vi "energie.vi"() -> ()   [LabVIEW 2024]
uses:
  <vilib>/Analysis/baseanly.llb/Mean (DBL).vi
  EFmeter.lvlib
  <vilib>/Analysis/NI_AALBase.lvlib
  BK Precision 8500B Series/BK Precision 8500B Series.lvlib
panel:
  in  "VISA resource name":refnum<visa-resource-name>
  in  "Clear":bool
  in  "Typ zatěže":u16(ring) items=["Manualni", "BK 8542B"]
  in  "Uložit data":bool
  in  "file path (use dialog)":path
  in  "Vzorku na krokù":u16 max=100 step=1
  in  "Prumerovani":bool
  in  "start":dbl
  out "error out 2":errorcluster
  in  "velikost kroku":dbl
  in  "VISA resource name 2":refnum<visa-resource-name>
  out "Aktuální Zátěž":dbl=2.5
  in  "Prodleva mezi vzorky":u32
  out "R_out":dbl
  in  "Pocet kroku":i32
  out "XY Graph 2":cluster{"X":dbl[], "Y":dbl[]}[](graph)
  in  "stop":bool
  in  "Start":bool
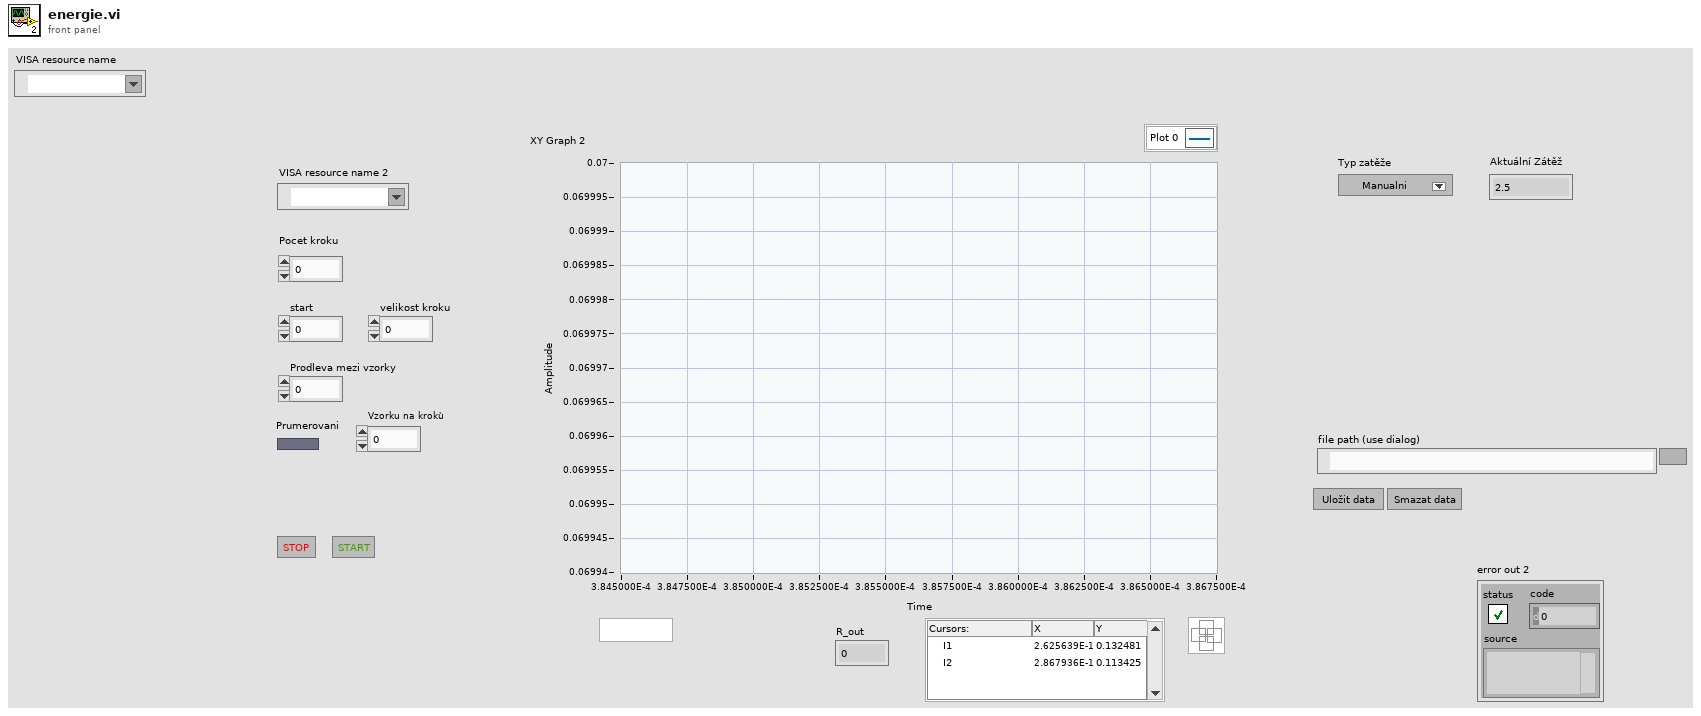
[diagram p1: front panel]
types:
  T1 = enum16{"init", "wait", "graph", "meas", "change_load", "init_measurment", "save", "clear"}
  T2 = typedef "LVCursorListTypeDef.ctl" = cluster{"Name":string, "Color":u32, "Style":u8, "Point Style":u8, "Name Visible":bool, "Allow Drag":bool, "Cursor Mode":u32, "Plot":i32, "Index":i32, "Position":cluster{"X":dbl, "Y":dbl}, "X Scale":u32, "Y Scale":u32, "Watch Plots":i32[], "Watch All Plots":bool, "Plot Area":i32, "Label Offset":cluster{"X":dbl, "Y":dbl}}[]
  T3 = cluster{"Name":string, "Color":u32, "Style":u8, "Point Style":u8, "Name Visible":bool, "Allow Drag":bool, "Cursor Mode":u32, "Plot":i32, "Index":i32, "Position":cluster{"X":dbl, "Y":dbl}, "X Scale":u32, "Y Scale":u32, "Watch Plots":i32[], "Watch All Plots":bool, "Plot Area":i32, "Label Offset":cluster{"X":dbl, "Y":dbl}}
  T4 = enum16{"open", "replace", "create", "open or create", "replace or create", "replace or create with confirmation"}
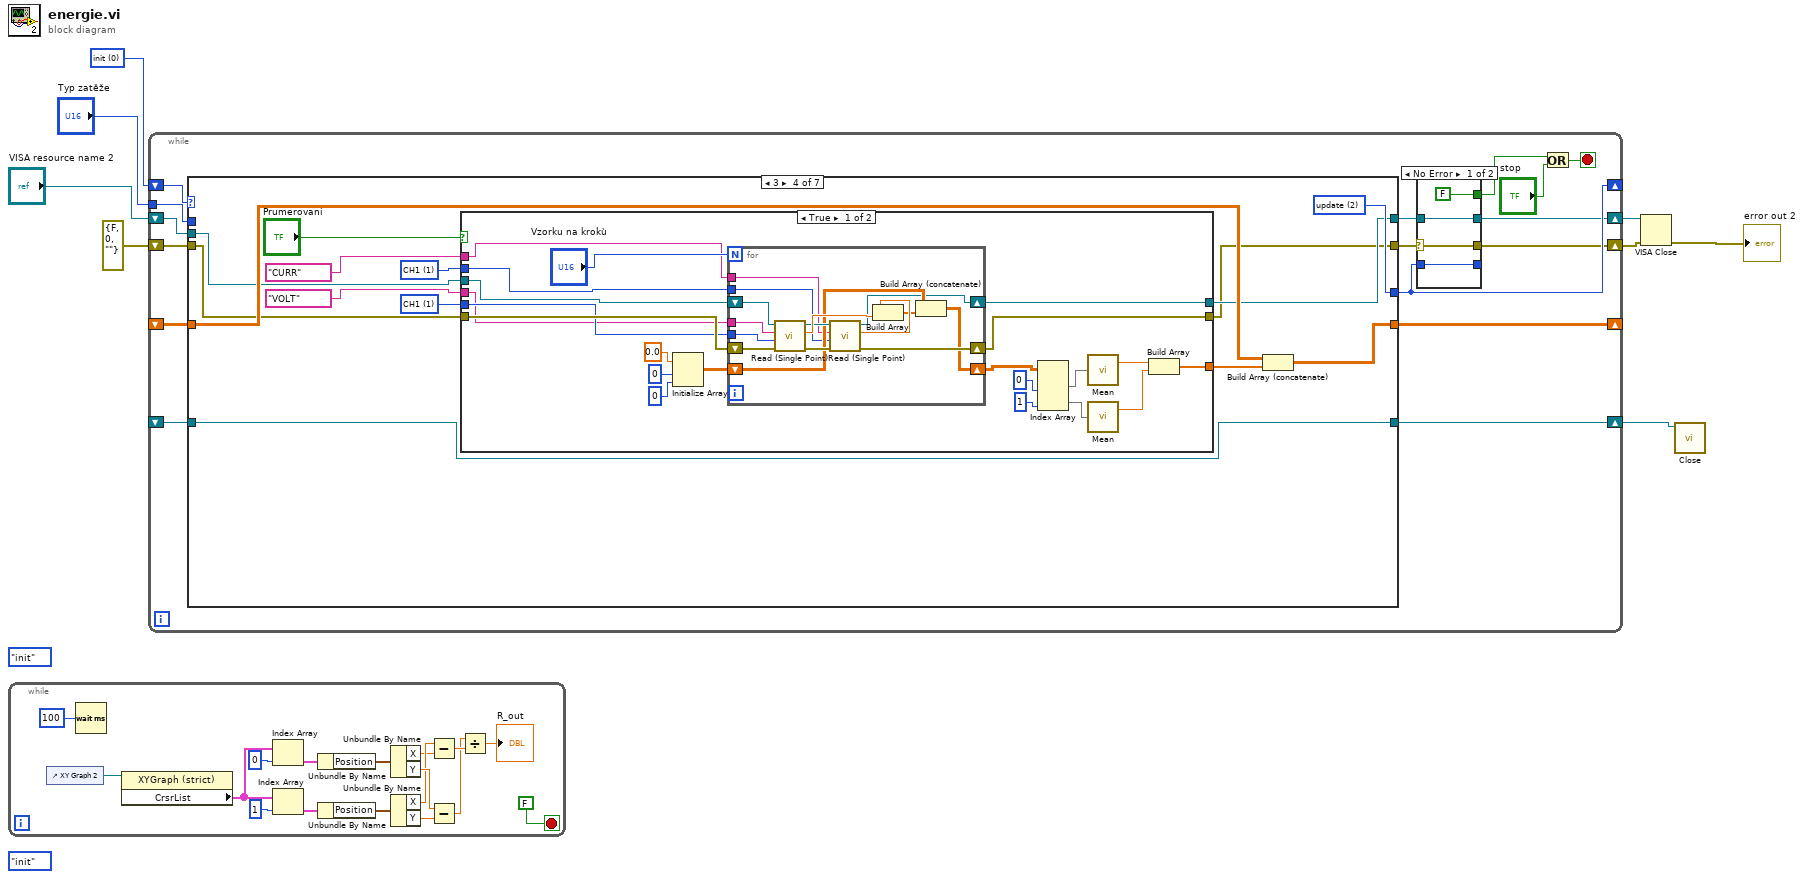
[diagram p0: block diagram]
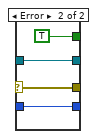
[diagram p2: hidden frame]
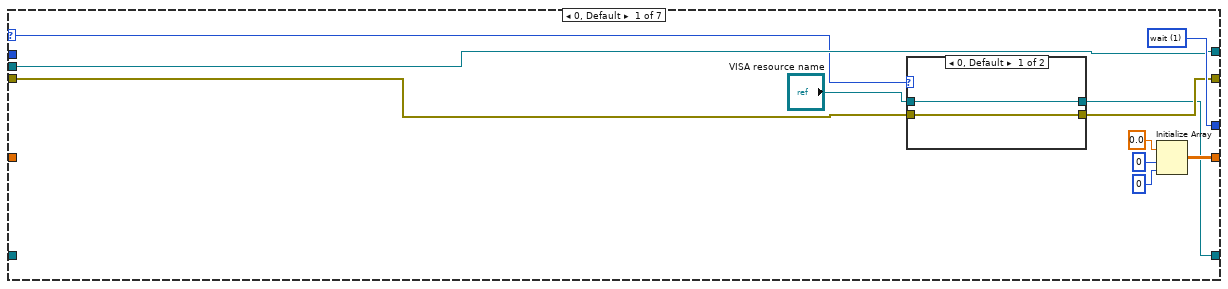
[diagram p3: hidden frame]
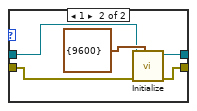
[diagram p4: hidden frame]
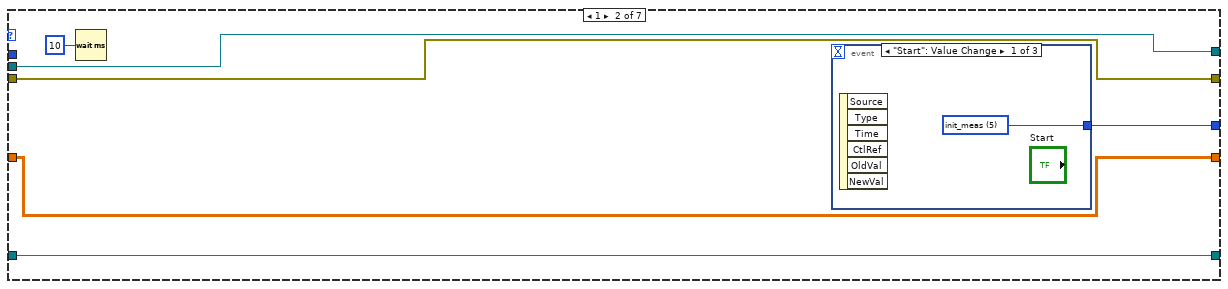
[diagram p5: hidden frame]
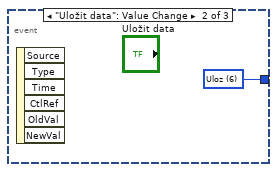
[diagram p6: hidden frame]
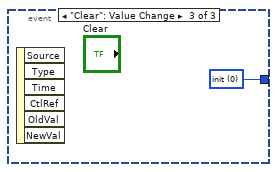
[diagram p7: hidden frame]
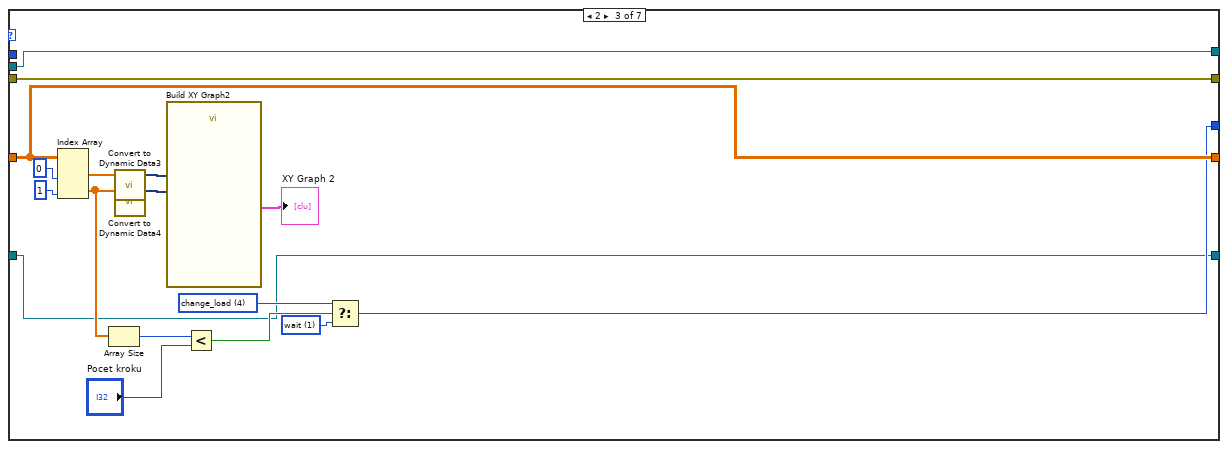
[diagram p8: hidden frame]
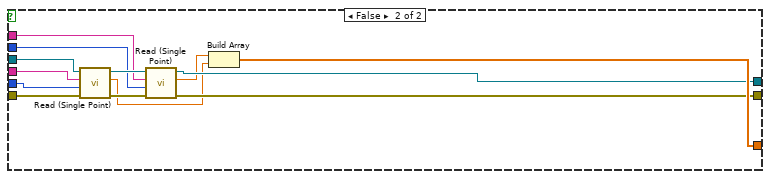
[diagram p9: hidden frame]
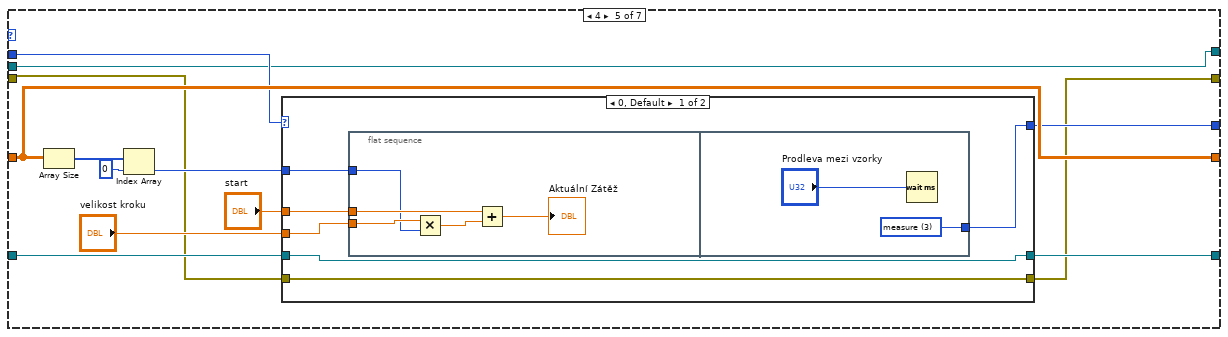
[diagram p10: hidden frame]
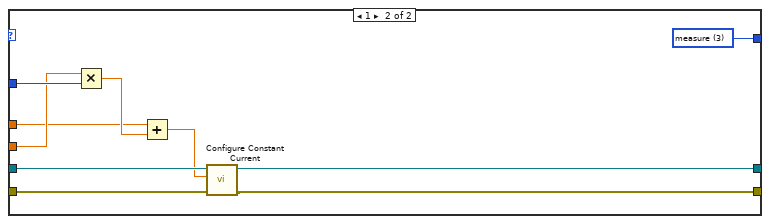
[diagram p11: hidden frame]
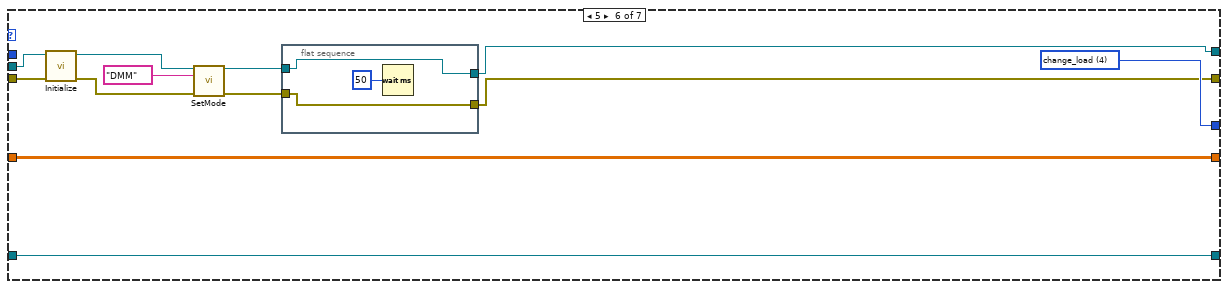
[diagram p12: hidden frame]
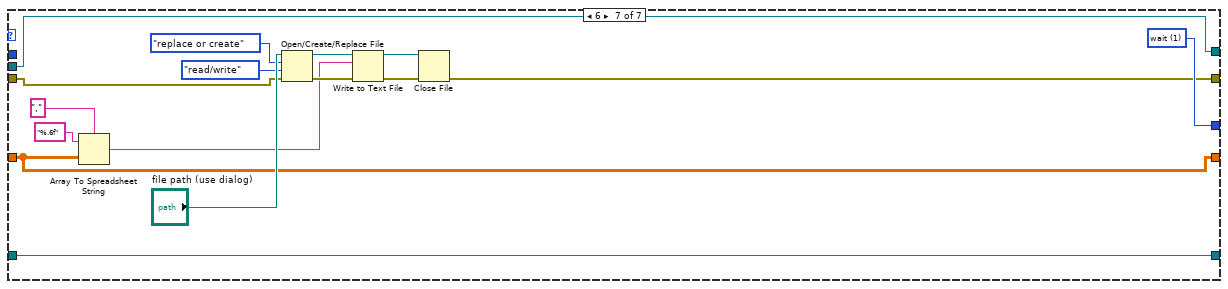
[diagram p13: hidden frame]
diagram:
  (unwired) T1."init"
  (unwired) T1."init"
  w8 = u16 0 items=["init", "wait", "update", "measure", "change_load", "init_meas", "Uloz", "clear"]
  n1 = while {
    stop <- FALSE stop-if-true
    n2 = control-ref of="XY Graph 2"() -> (w23:refnum<vi>)
    n3 = Wait (ms)(milliseconds to wait=u32 100) -> ()  [unwired: 1 out]
    n4 = property class="XYGraph (strict)"(reference=w23) -> ("CrsrList"=w18:T2)  [unwired: 1 in, 2 out]
    n5 = Index Array(array=w18, index=0) -> (element=w24:T3)
    n6 = Index Array(array=w18, index=1) -> (element=w20:T3)
    n7 = Unbundle By Name(w24) -> ("Position"=w25:cluster{"X":dbl, "Y":dbl})
    n8 = Unbundle By Name(w20) -> ("Position"=w21:cluster{"X":dbl, "Y":dbl})
    n9 = Unbundle By Name(w25) -> ("X"=w9:dbl, "Y"=w16:dbl)
    n10 = Unbundle By Name(w21) -> ("X"=w10:dbl, "Y"=w17:dbl)
    n11 = Subtract(x=w10, y=w9) -> (x-y=w12:dbl)
    n12 = Subtract(x=w16, y=w17) -> (x-y=w11:dbl)
    n13 = Divide(x=w11, y=w12) -> (x/y=→"R_out":dbl)
  }
  n14 = while {
    shift-right: [w41] -> _
    shift-left: _ -> [w40]
    shift-right: [w36] -> _
    shift-left: w8 -> [w39]
    shift-right: [w33] -> w4
    shift-left: "VISA resource name 2" -> [w38]
    shift-right: [w32] -> w3
    shift-left: errorcluster {"status"=FALSE, "code"=0, "source"=""} ("error in (no error)") -> [w37]
    tunnel: "Typ zatěže" -> [w28]
    shift-right: [w27] -> w1
    shift-left: _ -> [w26]
    stop <- w30 stop-if-true
    n15 = case shown="3" w39 {
      selector: w39 -> [w54 _ _ _ _ _ _]
      tunnel: [w58 w72 w85 w106 w169 w204 w218] -> w41
      tunnel: w40 -> [_ w72 w85 w107 w169 w204 w218]
      tunnel: [w57 w73 w84 w104 w167 w198 w216] -> w36
      tunnel: [w52 w70 w78 w96 w157 w195 w212] -> w35
      tunnel: [w55 w71 w79 w97 w166 w197 w223] -> w34
      tunnel: w38 -> [w55 w71 w79 w103 w166 w200 w223]
      tunnel: w37 -> [w53 w70 w78 w102 w158 w199 w219]
      tunnel: w28 -> [_ _ _ _ w168 _ _]
      tunnel: [w51 w68 w77 w94 w164 w193 w208] -> w27
      tunnel: w26 -> [_ w68 w77 w94 w165 w193 w208]
      frame 0, Default {
        w57 = u16 1 items=["init", "wait", "update", "measure"]
        n16 = case shown="0, Default" w54 {
          tunnel: w53 -> [w62 w66]
          tunnel: [w62 w65] -> w52
          tunnel: [w61 w64] -> w51
          tunnel: "VISA resource name" -> [w61 w63]
          frame 0, Default {
          }
          frame 1 {
            n17 = call "Initialize.vi"("Serial Configuration"=cluster{"Baud Rate":u32} {"Baud Rate"=9600}, "error in (no error)"=w66, "VISA resource name"=w63) -> ("error out"=w65:errorcluster, "VISA resource name out"=w64:refnum<visa-resource-name>)  [unwired: 7 in]
          }
        }
        n18 = Initialize Array(0.0 ("element"), 0 ("dimension size"), 0 ("dimension size")) -> (w58:dbl[][])
      }
      frame 1 {
        n19 = Wait (ms)(milliseconds to wait=u32 10) -> ()  [unwired: 1 out]
        n20 = event shown="[0] \"Start\": Value Change" {
          selector: _ -> [_ _ _]
          dyn-events: _ -> [_ _ _]
          timeout: _ -> [_ _ _]
          tunnel: [w74 w75 w76] -> w73
          event "Start": Value Change {
            w74 = u16 5 items=["init", "wait", "update", "measure", "change_load", "init_meas"]
            n21 = event-data() -> ()  [unwired: 1 in, 6 out]
          }
          event "Uložit data": Value Change {
            w75 = u16 6 items=["init", "wait", "update", "measure", "change_load", "init_meas", "Uloz"]
            n22 = event-data() -> ()  [unwired: 1 in, 6 out]
          }
          event "Clear": Value Change {
            w76 = u16 0 items=["init", "wait", "update", "measure", "change_load", "init_meas", "Uloz", "clear"]
            n23 = event-data() -> ()  [unwired: 1 in, 6 out]
          }
        }
      }
      frame 2 {
        w80 = u16 4 items=["init", "wait", "update", "measure", "change_load", "init_meas"]
        w86 = u16 1 items=["init", "wait", "update", "measure"]
        n24 = Index Array(array=w85, index (col) #1=0 ("index (row)"), index (col) #2=1 ("index (row)")) -> (element #1=w93:dbl[], element #2=w88:dbl[])  [unwired: 2 in]
        n25 = Array Size(array=w88) -> (size(s)=w90:i32)
        n26 = call "Convert to Dynamic Data3"("Array"=w93) -> ("Dynamic Data Type"=w92:dynamicdata)  [unwired: 3 in]
        n27 = call "Convert to Dynamic Data4"("Array"=w88) -> ("Dynamic Data Type"=w91:dynamicdata)  [unwired: 3 in]
        n28 = call "Build XY Graph2"("Y Input"=w91, "X Input"=w92) -> ("XY Graph"=→"XY Graph 2":cluster{"X":dbl[], "Y":dbl[]}[])  [unwired: 8 in, 1 out]
        n29 = Less?(x=w90, y="Pocet kroku") -> (x < y?=w89:bool)
        n30 = Select(t=w80, s=w89, f=w86) -> (s? t:f=w84:u16)
      }
      frame 3 {
        w98 = u16 1 items=["CH2"=2, "CH1"=1] ("Ring")
        w101 = u16 1 items=["CH2"=2, "CH1"=1] ("Ring")
        w104 = u16 2 items=["init", "wait", "update", "measure"]
        n31 = case shown="True" "Prumerovani" {
          tunnel: [w110 w156] -> w105
          tunnel: w103 -> [w123 w155]
          tunnel: w102 -> [w122 w154]
          tunnel: w101 -> [w121 w153]
          tunnel: "VOLT" ("Combo Box") -> [w120 w152]
          tunnel: "CURR" ("Combo Box") -> [w119 w149]
          tunnel: w98 -> [w118 w148]
          tunnel: [w109 w147] -> w97
          tunnel: [w108 w146] -> w96
          frame True {
            n32 = Initialize Array(0.0 ("element"), 0 ("dimension size"), 0 ("dimension size")) -> (w124:dbl[][])
            n33 = for {
              N: "Vzorku na krokù" -> [_]
              shift-right: [w136] -> w109
              shift-left: w123 -> [w137]
              shift-right: [w134] -> w108
              shift-left: w122 -> [w135]
              tunnel: w121 -> [w133]
              tunnel: w120 -> [w132]
              tunnel: w119 -> [w131]
              tunnel: w118 -> [w130]
              shift-right: [w129] -> w117
              shift-left: w124 -> [w138]
              n34 = call "Read (Single Point).vi"("error in (no error)"=w135, "Ring"=w133, "Combo Box"=w132, "VISA resource name"=w137) -> ("error out"=w141:errorcluster, "Measurement"=w143:dbl, "VISA resource name out"=w142:refnum<visa-resource-name>)  [unwired: 5 in]
              n35 = call "Read (Single Point).vi"("error in (no error)"=w141, "Ring"=w130, "Combo Box"=w131, "VISA resource name"=w142) -> ("error out"=w134:errorcluster, "Measurement"=w140:dbl, "VISA resource name out"=w136:refnum<visa-resource-name>)  [unwired: 5 in]
              n36 = Build Array(w140, w143) -> (w139:dbl[])
              n37 = Build Array (concatenate)(w138, w139) -> (w129:dbl[][])
            }
            n38 = Index Array(array=w117, index (col) #1=0 ("disabled index (col)"), index (col) #2=1 ("index (col)")) -> (element #1=w116:dbl[], element #2=w115:dbl[])  [unwired: 2 in]
            n39 = call-poly <vilib>:"Mean.vi"("X"=w116) -> ("mean"=w112:dbl)  [unwired: 1 out]
            n40 = call-poly <vilib>:"Mean.vi"("X"=w115) -> ("mean"=w111:dbl)  [unwired: 1 out]
            n41 = Build Array(w112, w111) -> (w110:dbl[])
          }
          frame False {
            n42 = call "Read (Single Point).vi"("error in (no error)"=w154, "Ring"=w153, "Combo Box"=w152, "VISA resource name"=w155) -> ("error out"=w151:errorcluster, "Measurement"=w144:dbl, "VISA resource name out"=w150:refnum<visa-resource-name>)  [unwired: 5 in]
            n43 = call "Read (Single Point).vi"("error in (no error)"=w151, "Ring"=w148, "Combo Box"=w149, "VISA resource name"=w150) -> ("error out"=w146:errorcluster, "Measurement"=w145:dbl, "VISA resource name out"=w147:refnum<visa-resource-name>)  [unwired: 5 in]
            n44 = Build Array(w145, w144) -> (w156:dbl[])
          }
        }
        n45 = Build Array (concatenate)(w107, w105) -> (w106:dbl[][])
      }
      frame 4 {
        n46 = Array Size(array=w169) -> (size(s)=w159:i32[])
        n47 = Index Array(array=w159, index=0) -> (element=w161:i32)
        n48 = case shown="0, Default" w168 {
          tunnel: [w175 w192] -> w167
          tunnel: w165 -> [w174 w191]
          tunnel: [w174 w190] -> w164
          tunnel: "velikost kroku" -> [w173 w188]
          tunnel: "start" -> [w172 w186]
          tunnel: w161 -> [w171 w189]
          tunnel: w158 -> [w170 w184]
          tunnel: [w170 w183] -> w157
          frame 0, Default {
            n49 = flat-sequence {
              tunnel: w173 -> [w178]
              tunnel: w172 -> [w177]
              tunnel: w171 -> [w176]
              tunnel: [w181] -> w175
              frame #0 {
                n50 = Multiply(x=w178, y=w176) -> (x*y=w180:dbl)
                n51 = Add(x=w177, y=w180) -> (x+y=→"Aktuální Zátěž":dbl)
              }
              frame #1 {
                w181 = u16 3 items=["init", "wait", "update", "measure", "change_load", "init_meas"]
                n52 = Wait (ms)(milliseconds to wait="Prodleva mezi vzorky") -> ()  [unwired: 1 out]
              }
            }
          }
          frame 1 {
            w192 = u16 3 items=["init", "wait", "update", "measure", "change_load", "init_meas"]
            n53 = Multiply(x=w188, y=w189) -> (x*y=w187:dbl)
            n54 = Add(x=w186, y=w187) -> (x+y=w185:dbl)
            n55 = call "Configure Constant Current.vi"("error in (no error)"=w184, "CC Current (0)"=w185, "VISA resource name"=w191) -> ("error out"=w183:errorcluster, "VISA resource name out"=w190:refnum<visa-resource-name>)  [unwired: 7 in]
          }
        }
      }
      frame 5 {
        w198 = u16 4 items=["init", "wait", "update", "measure", "change_load", "init_meas"]
        n56 = call "Initialize.vi"("error in (no error)"=w199, "VISA resource name"=w200) -> ("error out"=w203:errorcluster, "VISA resource name out"=w202:refnum<visa-resource-name>)  [unwired: 8 in]
        n57 = call "SetMode.vi"("VISA resource name"=w202, "Combo Box"="DMM", "error in (no error)"=w203) -> ("VISA resource name out"=w196:refnum<visa-resource-name>, "error out"=w194:errorcluster)  [unwired: 11 in]
        n58 = flat-sequence {
          tunnel: [w206] -> w197
          tunnel: w196 -> [w206]
          tunnel: w194 -> [w205]
          tunnel: [w205] -> w195
          frame #0 {
            n59 = Wait (ms)(milliseconds to wait=u32 50) -> ()  [unwired: 1 out]
          }
        }
      }
      frame 6 {
        w216 = u16 1 items=["init", "wait", "update", "measure", "change_load", "init_meas"]
        n60 = Array To Spreadsheet String(delimiter (Tab)=",", array=w218, 3:"%.6f" ("format string")) -> (spreadsheet string=w209:string)
        n61 = Open/Create/Replace File(file path (use dialog)="file path (use dialog)", error in=w219, operation (0:open)=T4."replace or create", access (0:read/write)=enum16{"read/write", "read-only", "write-only"}."read/write") -> (refnum out=w211:refnum<file>, error out=w214:errorcluster)  [unwired: 2 in, 1 out]
        n62 = Write to Text File(file (use dialog)=w211, text=w209, error in=w214) -> (refnum out=w210:refnum<file>, error out=w213:errorcluster)  [unwired: 1 in, 1 out]
        n63 = Close File(refnum=w210, error in=w213) -> (error out=w212:errorcluster)  [unwired: 1 out]
      }
    }
    n64 = case shown="No Error" w35 {
      selector: w35 -> [w43 w47]
      tunnel: w36 -> [w45 w48]
      tunnel: [w45 w48] -> _
      tunnel: w34 -> [w44 w49]
      tunnel: [w44 w49] -> w33
      tunnel: [w43 w47] -> w32
      tunnel: [FALSE TRUE] -> w29
      frame No Error {
      }
      frame Error {
      }
    }
    n65 = Or(x=w29, y="stop") -> (x .or. y?=w30:bool)
  }
  n66 = VISA Close(VISA resource name=w4, error in (no error)=w3) -> (error out=→"error out 2":errorcluster)
  n67 = call "Close.vi"("VISA resource name"=w1) -> ()  [unwired: 10 in, 1 out]
